vi "Multi_FID_Calib_Prog.vi"() -> ()   [LabVIEW 2015]
uses:
  Anemometry Sub Vis/Controls/Post_Process.ctl
  Anemometry Sub Vis/Globals/Meas_global.vi
  Anemometry Sub Vis/Globals/Preference_global.vi
panel:
  in  "Tab Control":T1(tab)=enum."Cal Data"
  in  "Auto Rig Name?":bool
  in  "Rig Name":string="WT3"
  in  "Cal File Options":T2(ring)
  out "Current Cal Files":path[](array[path])=[path "/CentralDataCache/Projects/9999/Calibrations/KAG69/FID_BG_k_a.xls", path "/CentralDataCache/Projects/9999/Calibrations/KAG69/FID_S1_k_a.xls", path "/CentralDataCache/Projects/9999/Calibrations/KAG69/FID_S2_k_a.xls", path "/CentralDataCache/Projects/9999/Calibrations/KAG69/FID_S3_k_a.xls"]
  in  "No. Cal Gases":u8=2 min=2 max=5 step=1
  out "Cal Gas Labels":string[](array[string])=["Zero Gas", "Cal Gas 1"]
  out "Cal Data":dbl[][](array[numeric])=[[0.41875017330812625, 0.8159171683400928, 1.3243110544381125, 0.14095187184693714], [0.40338683870299974, 0.9505751801295901, 1.9496582326971748, 0.13254361035114925]]
  out "Ref Data":dbl[](array[numeric])=[0.0, 465.0]
  out "FID Cals":cluster{"X array":dbl[], "Y array":dbl[]}[](graph)=[{"X array"=[0.0, 465.0], "Y array"=[0.41875017330812625, 0.40338683870299974]}, {"X array"=[0.0, 465.0], "Y array"=[0.8159171683400928, 0.9505751801295901]}, {"X array"=[0.0, 465.0], "Y array"=[1.3243110544381125, 1.9496582326971748]}, {"X array"=[0.0, 465.0], "Y array"=[0.14095187184693714, 0.13254361035114925]}]
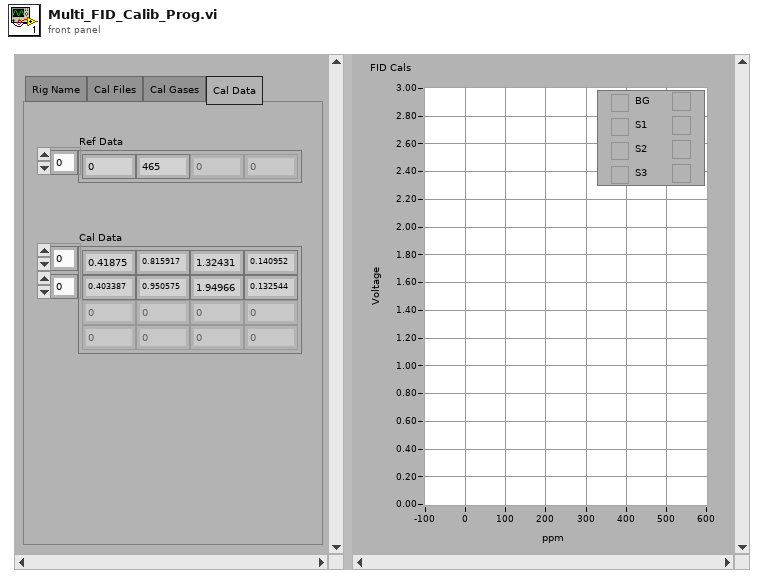
[diagram p1: front panel]
types:
  T1 = enum32{"Rig Name", "Cal Files", "Cal Gases", "Cal Data"}
  T2 = enum16{"New", "Add to Current", "Replace Current"}
  T3 = typedef "Post_Process.ctl" = enum16{"Take New Data", "Post Process Raw Data File"}
  T4 = typedef "Ch_description_ADAM.ctl" = cluster{"Ch Name":string, "Type":T5, "Function":T6, "Ch State":T7, "Calibration type":T8, "A":dbl, "B":dbl, "C":dbl, "D":dbl, "Comments":string, "Address":T9, "String":string, "Duty":u16}
  T5 = typedef "Module_type_ADAM.ctl" = string
  T6 = typedef "Function_ADAM.ctl" = enum16{"Analogue Input", "Digital Input", "Event counter", "Event rate", "Analogue Output", "Digital Output", "Relay Output"}
  T7 = typedef "Channel_State.ctl" = enum16{"On", "Off", "Always On", "Always Off"}
  T8 = typedef "Calib_type_ADAM.ctl" = enum16{"Raw", "Bx + A", "Cx^2 + Bx + A", "Dx^3 + Cx^2 + Bx + A", "In Band", "Hi-Tec Q", "Hi-Tec M_dot", "Text"}
  T9 = typedef "Address.ctl" = cluster{"Main":i32, "Ch.":i32, "Sub":i32, "Port Name":string}
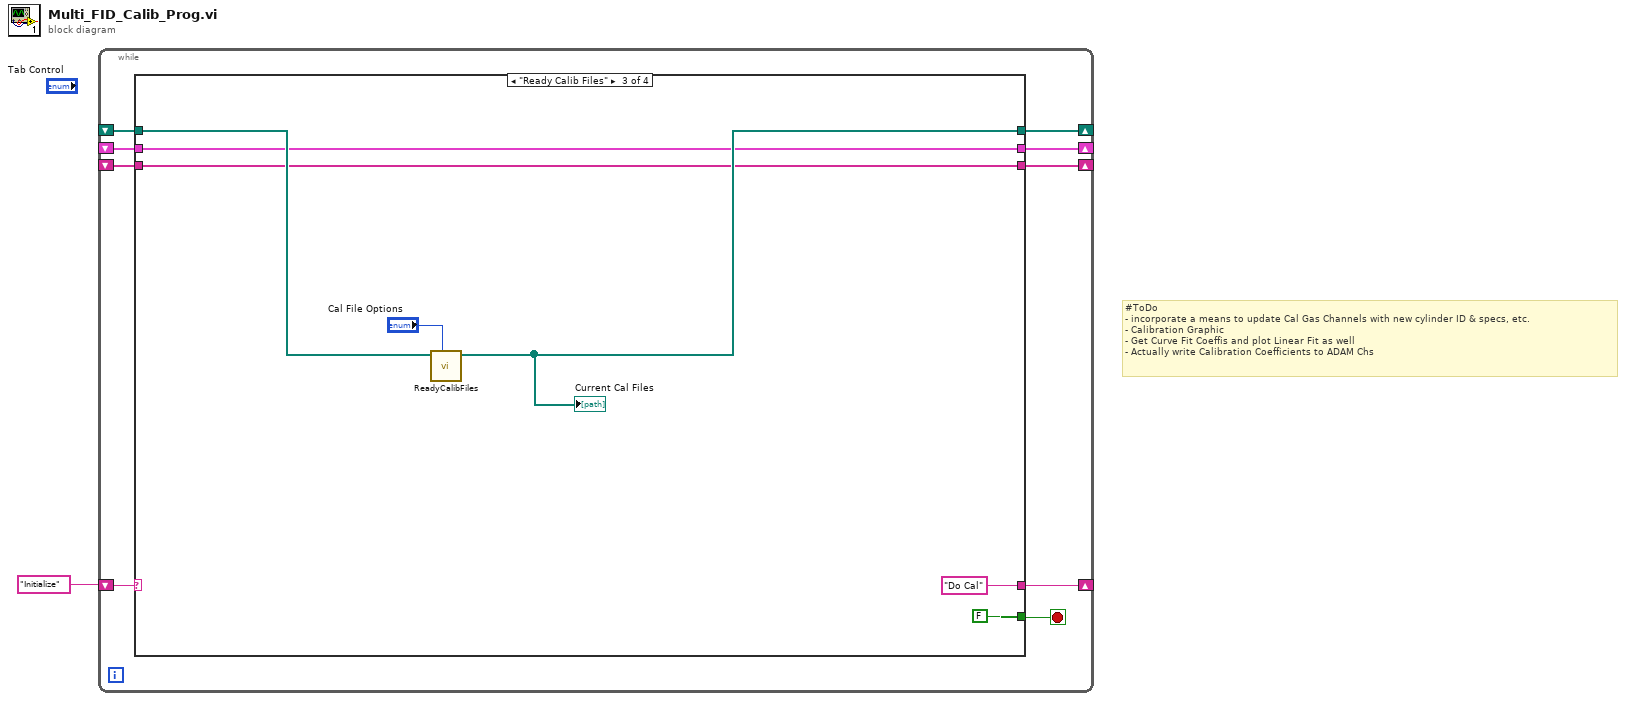
[diagram p0: block diagram]
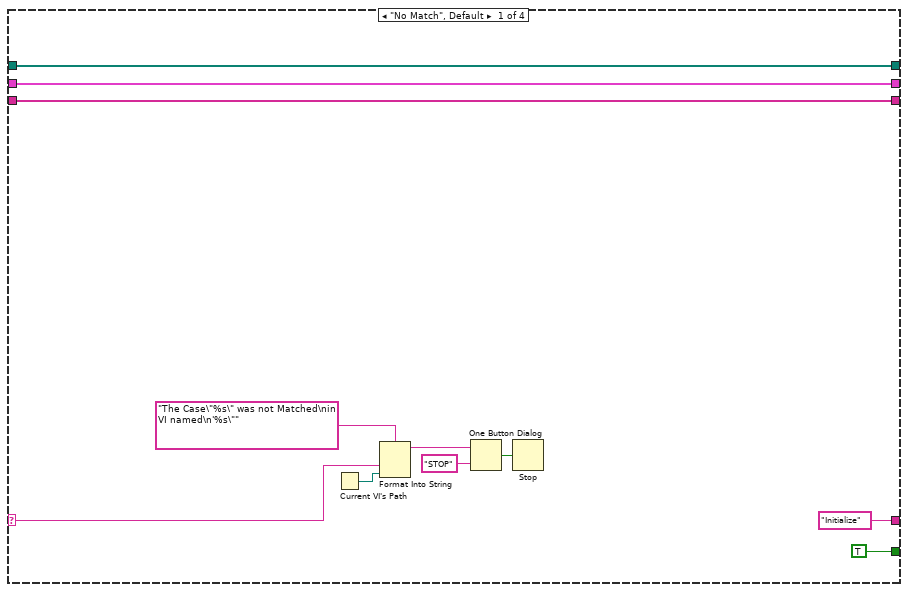
[diagram p2: hidden frame]
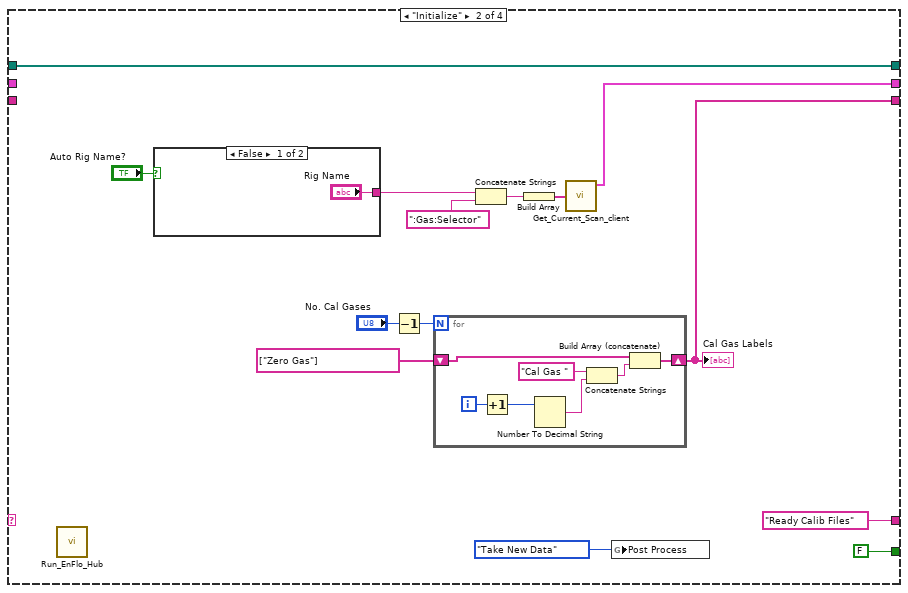
[diagram p3: hidden frame]
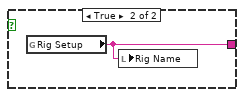
[diagram p4: hidden frame]
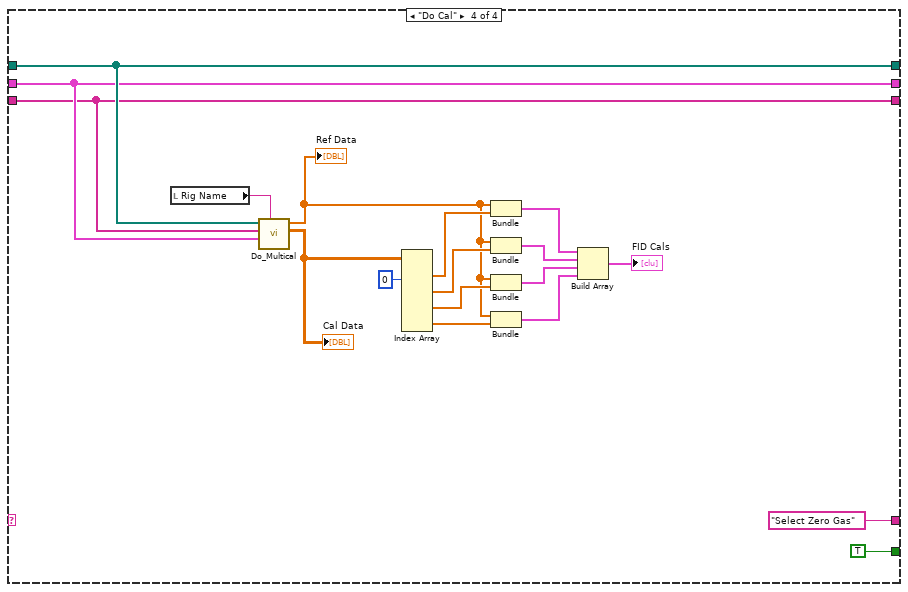
[diagram p5: hidden frame]
diagram:
  # "#ToDo\n- incorporate a means to update Cal Gas Channels with new cylinder ID & specs, etc.\n- Calibration Graphic\n- Get Curve Fit Coeffis and plot Linear Fit as well\n- Actually write Calibration Coefficients to ADAM Chs"
  n1 = while {
    shift-left: "Initialize" -> [w8]
    shift-right: [w9] -> _
    shift-right: [w7] -> _
    shift-left: _ -> [w6]
    shift-right: [w4] -> _
    shift-left: _ -> [w5]
    shift-right: [w3] -> _
    shift-left: _ -> [w2]
    stop <- w10 stop-if-true
    n2 = case shown="\"Ready Calib Files\"" w8 {
      selector: w8 -> [w11 _ _ _]
      tunnel: [TRUE FALSE FALSE TRUE] -> w10
      tunnel: ["Initialize" "Ready Calib Files" ("t") "Do Cal" ("t") "Select Zero Gas" ("t")] -> w9
      tunnel: [w14 w33 w48 w66] -> w7
      tunnel: w6 -> [w14 w33 w47 w66]
      tunnel: w5 -> [w13 _ w46 w65]
      tunnel: [w13 w23 w46 w65] -> w4
      tunnel: [w12 w29 w45 w64] -> w3
      tunnel: w2 -> [w12 _ w45 w64]
      frame "No Match", Default {
        n3 = Current VI's Path() -> (path=w16:path)
        n4 = Format Into String(format string="The Case\"%s\" was not Matched\nin VI named\n'%s\"" ("Format String"), w11, w16) -> (resulting string=w19:string)  [unwired: 2 in, 1 out]
        n5 = One Button Dialog(message=w19, button name ("OK")="STOP") -> (true=w17:bool)
        n6 = Stop(stop? (T)=w17) -> ()
      }
      frame "Initialize" {
        n7 = call "Run_EnFlo_Hub.vi"() -> ()  [unwired: 8 in]
        n8 = case shown="False" "Auto Rig Name?" {
          tunnel: ["Rig Name" w37] -> w27
          frame False {
          }
          frame True {
            n9 = global read "Preference_global.vi" "Rig Setup"() -> (w37:string)
            n10 = local write "Rig Name"(w37) -> ()
          }
        }
        n11 = Decrement(x="No. Cal Gases") -> (x-1=w30:u8)
        n12 = for {
          N: w30 -> [_]
          shift-right: [w43] -> w29
          shift-left: string[] ["Zero Gas"] -> [w44]
          i -> [w42]
          n13 = Increment(x=w42) -> (x+1=w41:i32)
          n14 = Number To Decimal String(number=w41) -> (decimal integer string=w39:string)  [unwired: 1 in]
          n15 = Concatenate Strings("Cal Gas ", w39) -> (w38:string)
          n16 = Build Array (concatenate)(w44, w38) -> (w43:string[])
        }
        "Cal Gas Labels" <- w29
        n17 = Concatenate Strings(w27, ":Gas:Selector") -> (w28:string)
        n18 = Build Array(w28) -> (w24:string[])
        n19 = call "Get_Current_Scan_client.vi"("ADAM Ch Names"=w24) -> ("Ch Description Array"=w23:T4[])  [unwired: 3 out]
        n20 = global write "Meas_global.vi" "Post Process"(Post_Process."Take New Data" ("Post Process")) -> ()
      }
      frame "Ready Calib Files" {
        n21 = call "ReadyCalibFiles.vi"("Cal File Options"="Cal File Options", "Calib Fnames IN"=w47) -> ("Calib Fnames OUT"=w48:path[])  [unwired: 9 in]
        "Current Cal Files" <- w48
      }
      frame "Do Cal" {
        n22 = local read "Rig Name"() -> (w67:string)
        n23 = call "Do_Multical.vi"("Rig Name"=w67, "Rig Gas Selector Ch"=w65, "Cal Gas Selection"=w64, "Calib Filepaths"=w66) -> ("Cal Data"=w63:dbl[][], "Ref Data"=w57:dbl[])  [unwired: 6 in]
        "Cal Data" <- w63
        "Ref Data" <- w57
        n24 = Index Array(array=w63, index (col) #1=0 ("disabled index (col)")) -> (element #1=w61:dbl[], element #2=w60:dbl[], element #3=w59:dbl[], element #4=w58:dbl[])  [unwired: 7 in]
        n25 = Bundle("Ref Data"=w57, "Cal Data"=w61) -> (w56:cluster{"Ref Data":dbl[], "Cal Data":dbl[]})  [unwired: 1 in]
        n26 = Bundle("Ref Data"=w57, "Cal Data"=w60) -> (w55:cluster{"Ref Data":dbl[], "Cal Data":dbl[]})  [unwired: 1 in]
        n27 = Bundle("Ref Data"=w57, "Cal Data"=w59) -> (w54:cluster{"Ref Data":dbl[], "Cal Data":dbl[]})  [unwired: 1 in]
        n28 = Bundle("Ref Data"=w57, "Cal Data"=w58) -> (w53:cluster{"Ref Data":dbl[], "Cal Data":dbl[]})  [unwired: 1 in]
        n29 = Build Array(w56, w55, w54, w53) -> (→"FID Cals":cluster{"Ref Data":dbl[], "Cal Data":dbl[]}[])
      }
    }
  }
